vi "new sweep.vi"() -> ()   [LabVIEW 2016, in "Lockin.DAQ.lvclass"]
uses:
  Lockin.DAQ.lvclass
  <vilib>/Analysis/1siggen.llb/Ramp Pattern by Samples.vi
  <vilib>/Analysis/NI_AALBase.lvlib
panel:
  in  "milliseconds to wait":u32
  out "XY Graph 2":cluster{"Ramp Pattern":dbl[], dbl[]}[](graph)
  in  "Back and forth ?":bool
  out "XY Graph":T1(graph)
  out "Numeric 2":i32
  out "Numeric 1":i32
  out "Numeric 3":i32
  in  "DC":dbl[](array[numeric])
  in  "Sweep Channel":i32[](array[numeric])
  in  "Sweep End (V)":dbl[](array[numeric])
  in  "Sweep Start (V)":dbl[](array[numeric])
  out "End (V)":dbl[](array[numeric])
  out "Start (V)":dbl[](array[numeric])
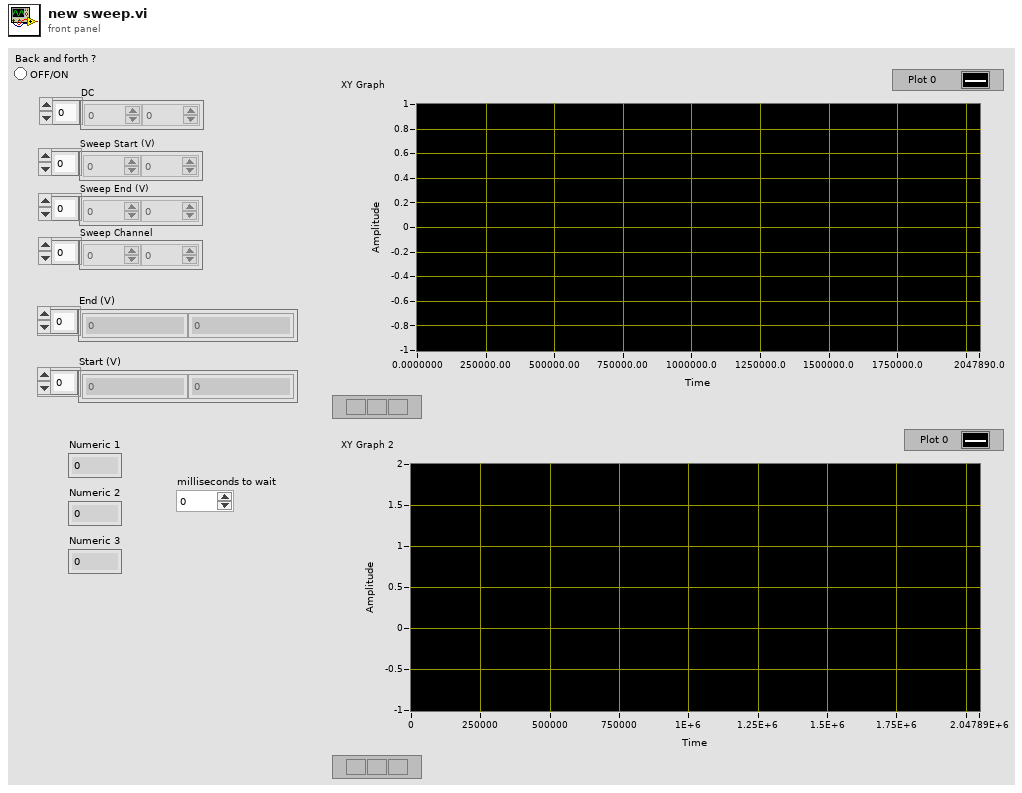
[diagram p1: front panel]
types:
  T1 = cluster{"Ramp Pattern":dbl[], "Ramp Pattern":dbl[]}[]
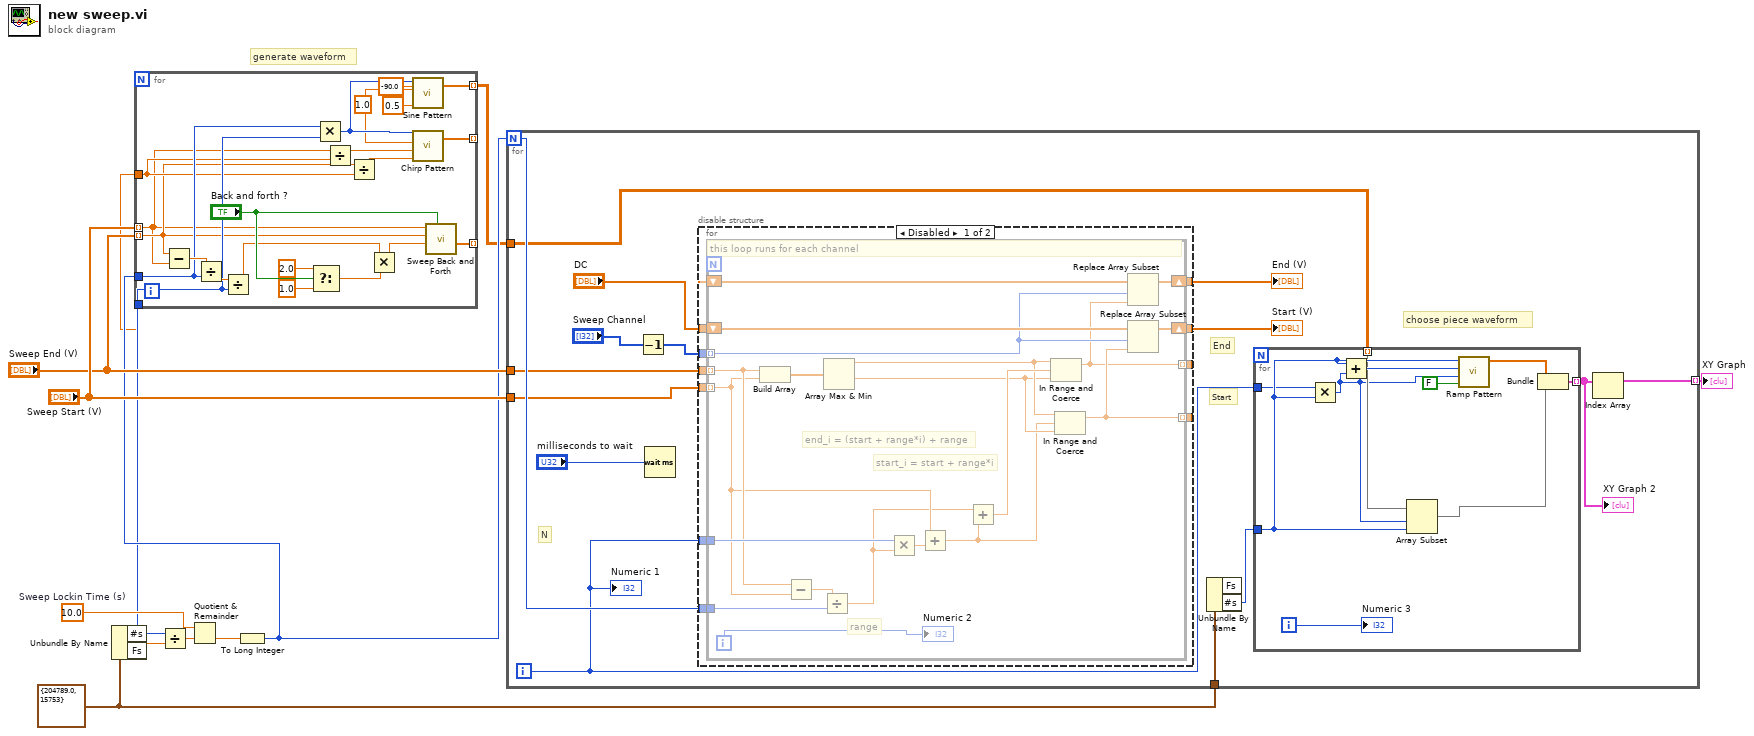
[diagram p0: block diagram]
diagram:
  w10 = 10.0  # Sweep Lockin Time (s)
  w8 = cluster{"Fs":dbl, "#s":i32} {"Fs"=204789.0, "#s"=15753} ("input cluster")
  # "generate waveform"
  n1 = Unbundle By Name(w8) -> ("#s"=w3:i32, "Fs"=w2:dbl)
  n2 = Divide(x=w3, y=w2) -> (x/y=w9:dbl)
  n3 = Quotient & Remainder(x=w10, y=w9) -> (floor(x/y)=w5:dbl)  [unwired: 1 out]
  n4 = To Long Integer(number=w5) -> (32bit integer=w4:i32)
  n5 = for {
    tunnel: "Sweep Start (V)" -> [w17] mode=indexing
    tunnel: "Sweep End (V)" -> [w18] mode=indexing
    tunnel: [w33] -> _ mode=indexing
    tunnel: w4 -> [w24]
    tunnel: w3 -> [w23]
    tunnel: [w22] -> _ mode=indexing
    tunnel: w2 -> [w19]
    tunnel: [w12] -> w1 mode=indexing
    w15 = 1.0 ("amplitude")
    n6 = Subtract(x=w18, y=w17) -> (x-y=w32:dbl)
    n7 = Divide(x=w32, y=w24) -> (x/y=w31:dbl)
    n8 = Divide(x=w31, y=w23) -> (x/y=w27:dbl)
    n9 = Select(t=2.0, s="Back and forth ?", f=1.0) -> (s? t:f=w29:dbl)
    n10 = Multiply(x=w24, y=w23) -> (x*y=w16:i32)
    n11 = Divide(x=w17, y=w19) -> (x/y=w21:dbl)
    n12 = Divide(x=w18, y=w19) -> (x/y=w20:dbl)
    n13 = Multiply(x=w27, y=w29) -> (x*y=w28:dbl)
    n14 = call <vilib>:"Sine Pattern.vi"("cycles"=0.5, "phase(degrees)"=-90.0, "amplitude"=w15, "samples"=w16) -> ("Sinusoidal Pattern"=w12:dbl[])  [unwired: 1 out]
    n15 = call <vilib>:"Chirp Pattern.vi"("f2"=w20, "f1"=w21, "amplitude"=w15, "samples"=w16) -> ("Chirp Pattern"=w22:dbl[])  [unwired: 1 out]
    n16 = call <userlib>:"Sweep Back and Forth.vi"("Back and forth ?"="Back and forth ?", "Step"=w28, "Final"=w18, "Initial"=w17) -> ("Output array"=w33:dbl[])  [unwired: 4 in, 2 out]
  }
  n17 = for {
    N: w4 -> [w42]
    tunnel: [w43] -> w11 mode=indexing
    tunnel: w8 -> [w41]
    tunnel: "Sweep Start (V)" -> [w39]
    tunnel: "Sweep End (V)" -> [w38]
    tunnel: w1 -> [w36]
    i -> [w40]
    # "choose piece waveform"
    # "Start"
    # "End"
    # "N"
    n18 = Decrement(x="Sweep Channel") -> (x-1=w48:i32[])
    n19 = Wait (ms)(milliseconds to wait="milliseconds to wait") -> ()  [unwired: 1 out]
    n20 = disable-structure shown="Disabled" {
      disable-tunnel: w48 -> [w58 _]
      disable-tunnel: "DC" -> [w57 _]
      disable-tunnel: [w56 _] -> w46
      disable-tunnel: [w55 _] -> w45
      disable-tunnel: [w54 _] -> _
      disable-tunnel: [w53 _] -> _
      disable-tunnel: w42 -> [w52 _]
      disable-tunnel: w40 -> [w51 _]
      disable-tunnel: w39 -> [w50 _]
      disable-tunnel: w38 -> [w49 _]
      frame Disabled {
        n21 = for {
          shift-right: [w77] -> w56
          shift-left: w57 -> [w78]
          shift-right: [w75] -> w55
          shift-left: w57 -> [w76]
          tunnel: w50 -> [w61] mode=indexing
          tunnel: w49 -> [w69] mode=indexing
          tunnel: w58 -> [w70] mode=indexing
          tunnel: w51 -> [w72]
          tunnel: w52 -> [w74]
          tunnel: [w65] -> w53 mode=indexing
          tunnel: [w64] -> w54 mode=indexing
          i -> [w60]
          # "end_i = (start + range*i) + range"
          # "start_i = start + range*i"
          # "range"
          # "this loop runs for each channel"
          n22 = Build Array(w69, w61) -> (w68:dbl[])
          n23 = Subtract(x=w69, y=w61) -> (x-y=w63:dbl)
          n24 = Divide(x=w63, y=w74) -> (x/y=w59:dbl)
          n25 = Array Max & Min(array=w68) -> (max value=w67:dbl, min value=w66:dbl)  [unwired: 2 out]
          n26 = Multiply(x=w72, y=w59) -> (x*y=w73:dbl)
          n27 = Add(x=w61, y=w73) -> (x+y=w62:dbl)
          n28 = Add(x=w59, y=w62) -> (x+y=w71:dbl)
          n29 = In Range and Coerce(upper limit=w67, x=w71, lower limit=w66) -> (coerced(x)=w64:dbl)  [unwired: 1 out]
          n30 = In Range and Coerce(upper limit=w67, x=w62, lower limit=w66) -> (coerced(x)=w65:dbl)  [unwired: 1 out]
          n31 = Replace Array Subset(array=w78, new element=w64, index=w70) -> (w77:dbl[])
          n32 = Replace Array Subset(array=w76, new element=w65, index=w70) -> (w75:dbl[])
          "Numeric 2" <- w60
        }
      }
      frame Enabled {
      }
    }
    "Start (V)" <- w45
    "End (V)" <- w46
    n33 = Unbundle By Name(w41) -> ("#s"=w44:i32)  [unwired: 1 out]
    n34 = for {
      tunnel: w44 -> [w87]
      tunnel: [w84] -> w34 mode=indexing
      tunnel: w40 -> [w83]
      tunnel: w36 -> [w81] mode=indexing
      i -> [w88]
      n35 = Multiply(x=w83, y=w87) -> (x*y=w80:i32)
      n36 = Add(x=w87, y=w80) -> (x+y=w86:i32)
      n37 = Array Subset(array=w81, index=w80, length=w87) -> (w79:dbl[])
      n38 = call-poly <vilib>:"Ramp Pattern.vi"("exclude end?"=FALSE, "start"=w80, "end"=w86, "samples"=w87) -> ("Ramp Pattern"=w85:dbl[])  [unwired: 6 in, 1 out]
      n39 = Bundle("Ramp Pattern"=w85, w79) -> (w84:cluster{"Ramp Pattern":dbl[], dbl[]})  [unwired: 1 in]
      "Numeric 3" <- w88
    }
    "XY Graph 2" <- w34
    n40 = Index Array(array=w34) -> (element=w43:cluster{"Ramp Pattern":dbl[], dbl[]})  [unwired: 1 in]
    "Numeric 1" <- w40
  }
  "XY Graph" <- w11
